vi "NI PXI Programmable Power Supply Ch Page.vi"(8 "error in (no error)":errorcluster, 11 "Node Ptr":T3 format="%.0x") -> (0 "error out":errorcluster)   [LabVIEW 2018, in "NI PXI-4110 Programmable Power Supply Custom Device.lvlib"]
uses:
  NI PXI-4110 Programmable Power Supply Custom Device.lvlib
  <vilib>/NI Veristand/Custom Device API/Custom Device Item Ref.ctl
  IO_Type.ctl
  4110_Channel #.ctl
  4110_Global.vi
  <vilib>/NI Veristand/Custom Device API/Get Item Property (Boolean).vi
  <vilib>/NI Veristand/Custom Device API/Get Item Property (U16).vi
  <vilib>/NI Veristand/Custom Device API/Get Item Property (Double).vi
  <vilib>/NI Veristand/Custom Device API/Set Item Property (U16).vi
  <vilib>/NI Veristand/Custom Device API/Set Item Property (Double).vi
  <vilib>/NI VeriStand/Custom Device API/Custom Device API.lvlib
panel:
  in  "Channel #":T1
  in  "Voltage Limit":dbl caption="Range (0-6V)" format="%.4f"
  in  "Initial Current Value":dbl caption="Range (0.01 -1A)" format="%.4f"
  in  "Current Limit":dbl caption="Range (0.01-1A)" format="%.4f"
  in  "IO Type":T2
  in  "Initial Voltage Value":dbl caption="Range (0-6V)" format="%_4f"
  in  "Name":string
  in  "Header":cluster{"Section Name":string}={"Section Name"="PXI-4110  Settings"}
  in  "Description":string
  # "Voltage  IO Settings"
  # "Current IO Settings"
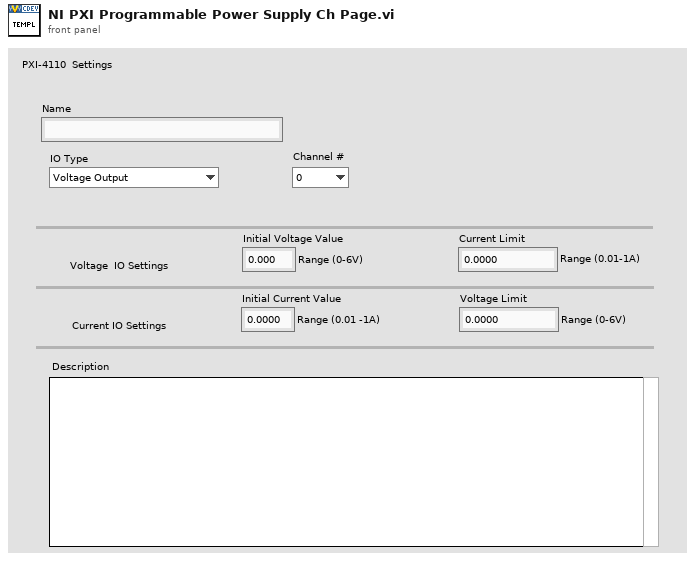
[diagram p1: front panel]
types:
  T1 = typedef "NI PXI-4110 Programmable Power Supply Custom Device.lvlib/4110_Channel #.ctl" = enum16{"0", "1", "2"}
  T2 = typedef "NI PXI-4110 Programmable Power Supply Custom Device.lvlib/IO_Type.ctl" = enum16{"Voltage Output", "Current Output"}
  T3 = typedef "Custom Device API.lvlib/Custom Device Item Ref.ctl" = u64
  T4 = cluster{"V_min":dbl, "V_max":dbl, "I_min":dbl, "I_max":dbl}
  T5 = enum8{"Enabled", "Disabled", "Disabled and Grayed Out"}
  T6 = typedef "Custom Device API.lvlib/Custom Device Item Info.ctl" = cluster{"Name":string, "Is Channel":bool, "GUID":string, "Is Waveform":bool}
  T7 = typedef "Custom Device API.lvlib/Custom Device Commands.ctl" = enum16{"Default", "Item renamed", "Shutdown", "Dynamic button pressed"}
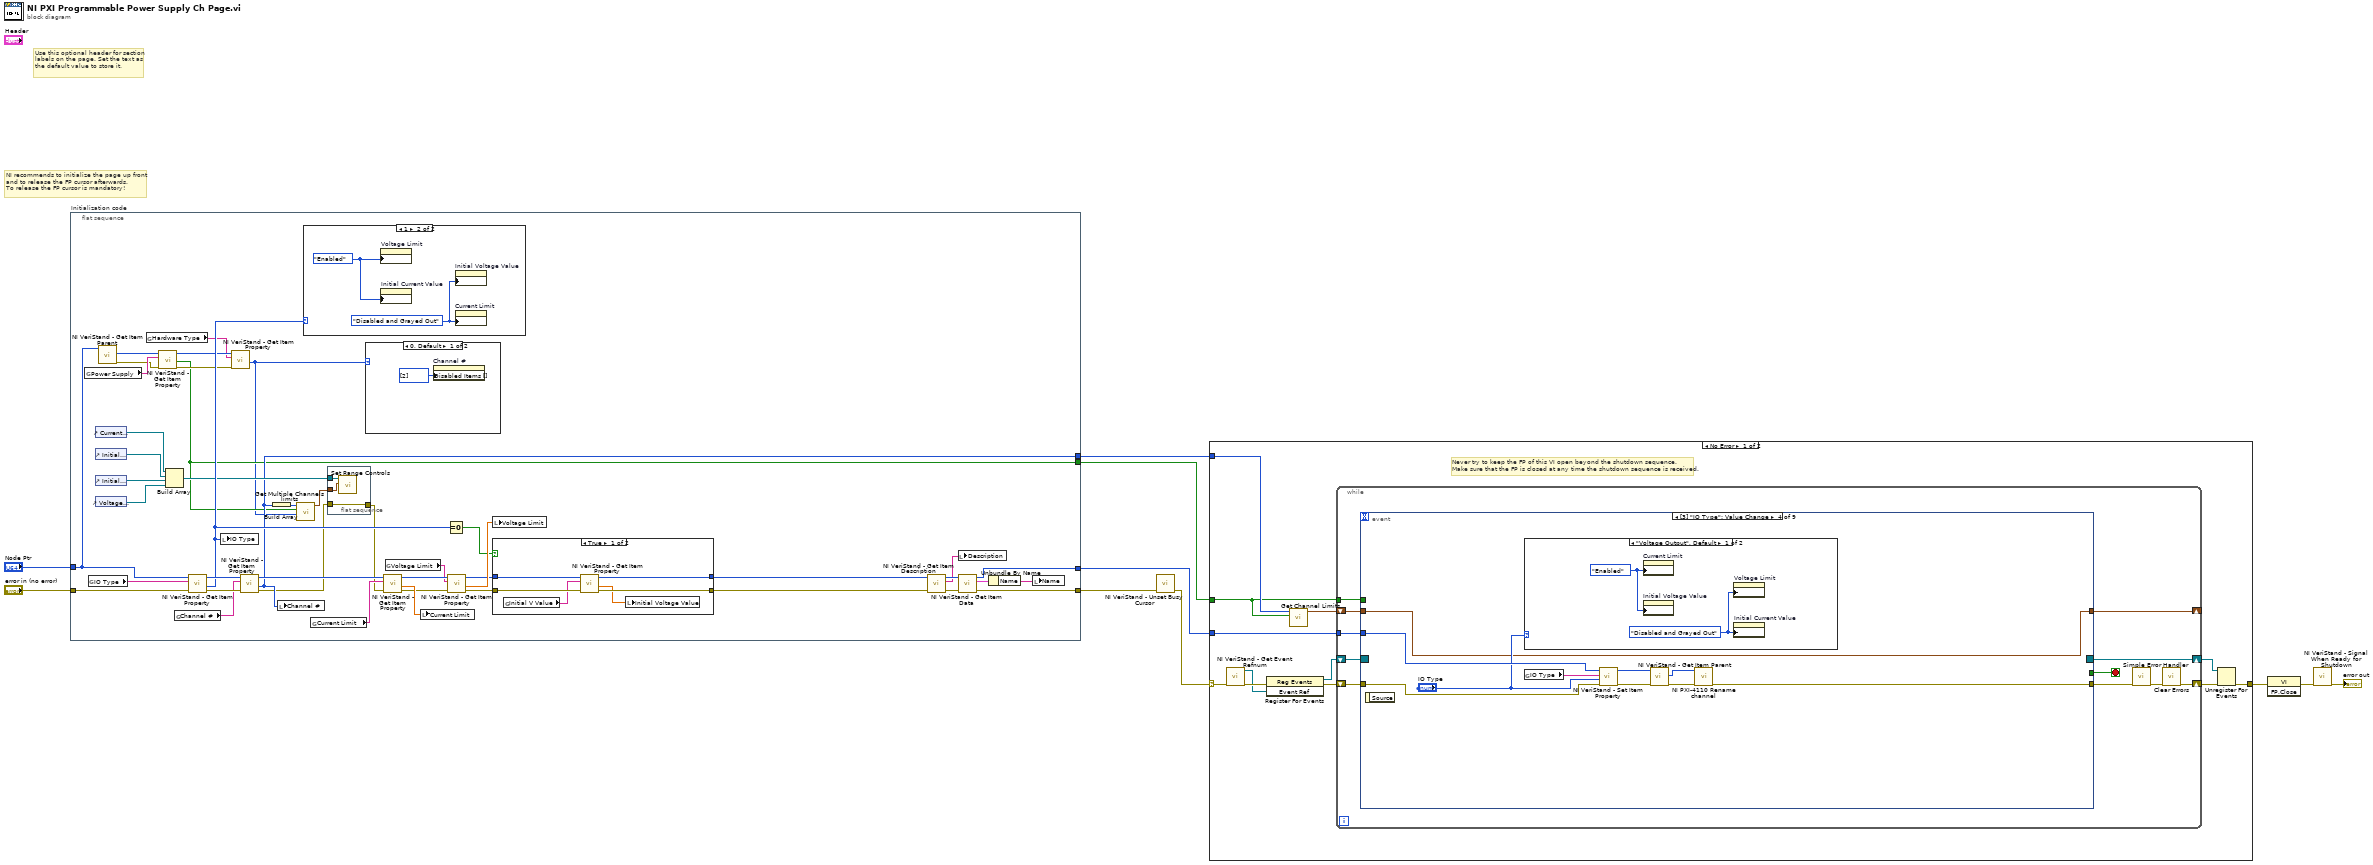
[diagram p0: block diagram]
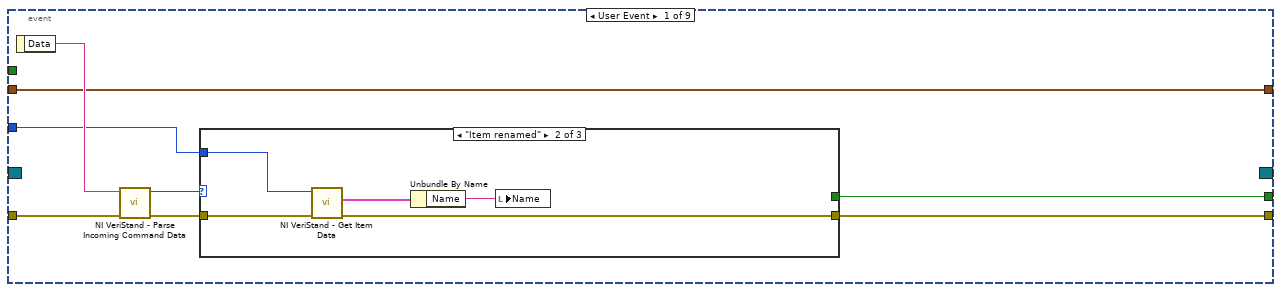
[diagram p2: hidden frame]
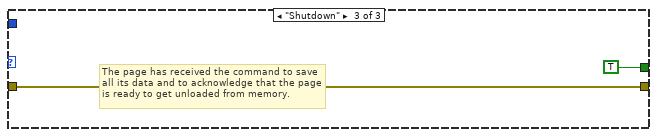
[diagram p4: hidden frame]
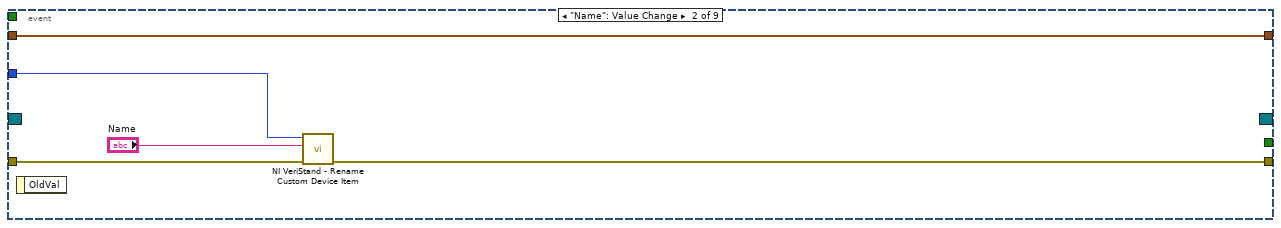
[diagram p5: hidden frame]
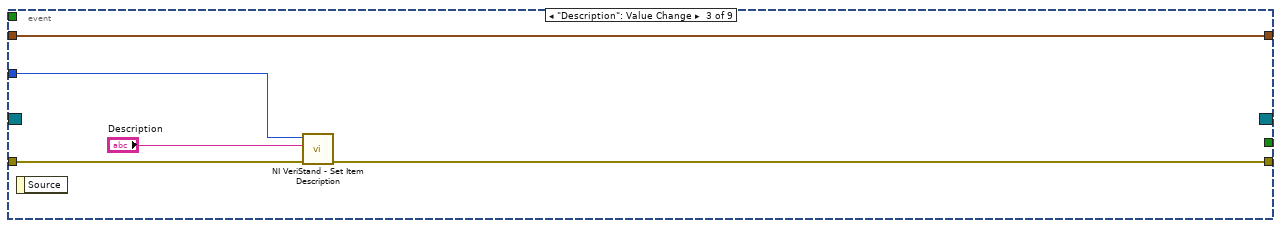
[diagram p6: hidden frame]
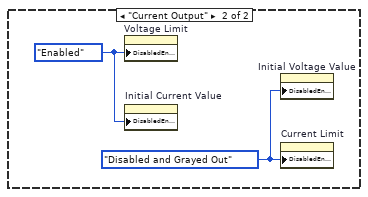
[diagram p7: hidden frame]
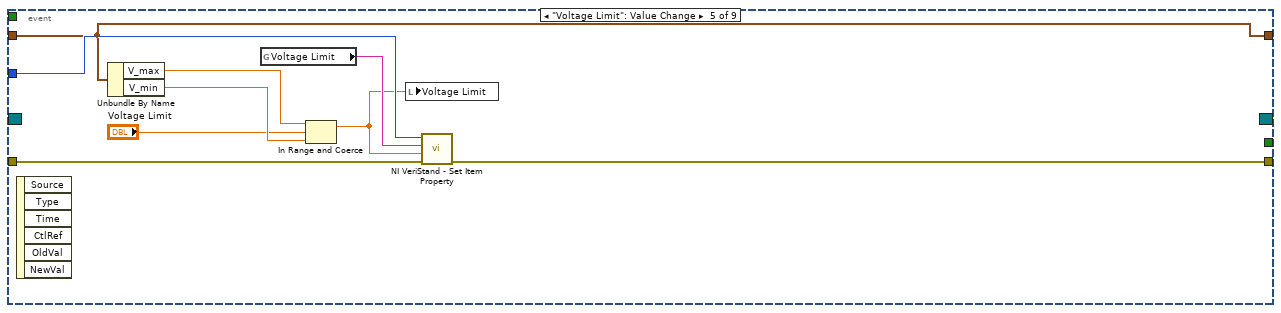
[diagram p8: hidden frame]
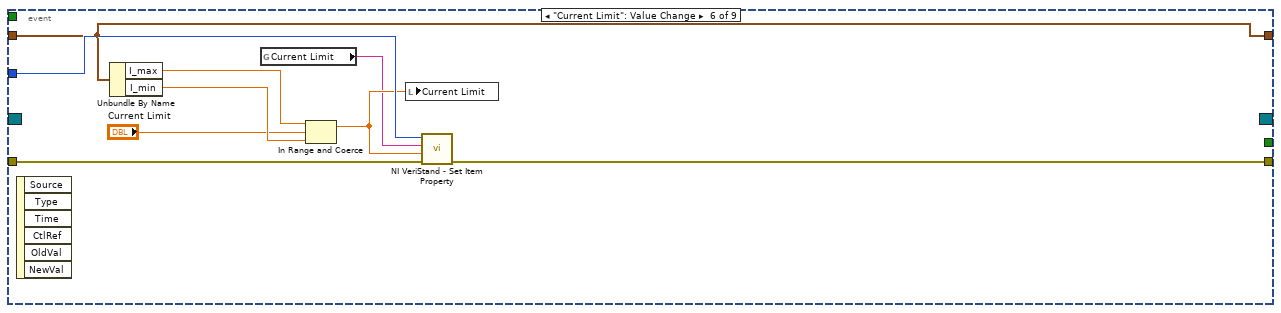
[diagram p9: hidden frame]
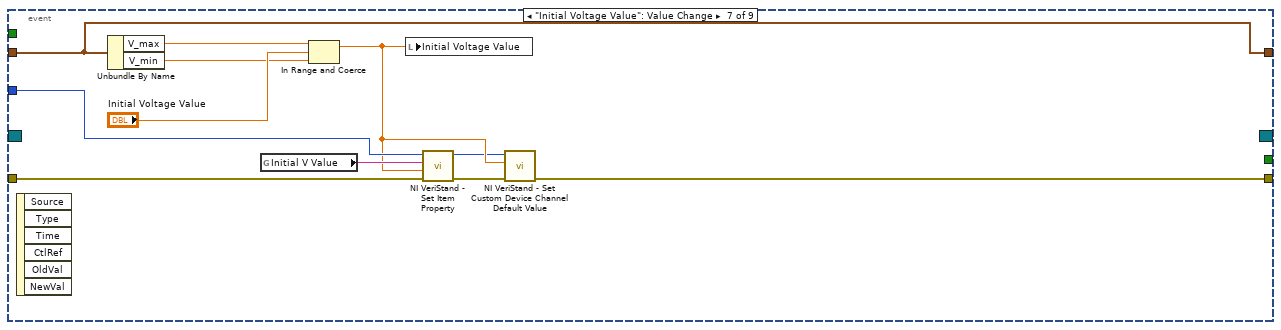
[diagram p10: hidden frame]
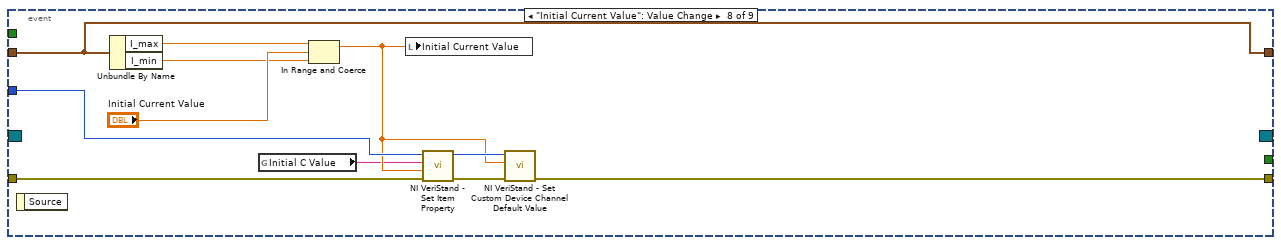
[diagram p11: hidden frame]
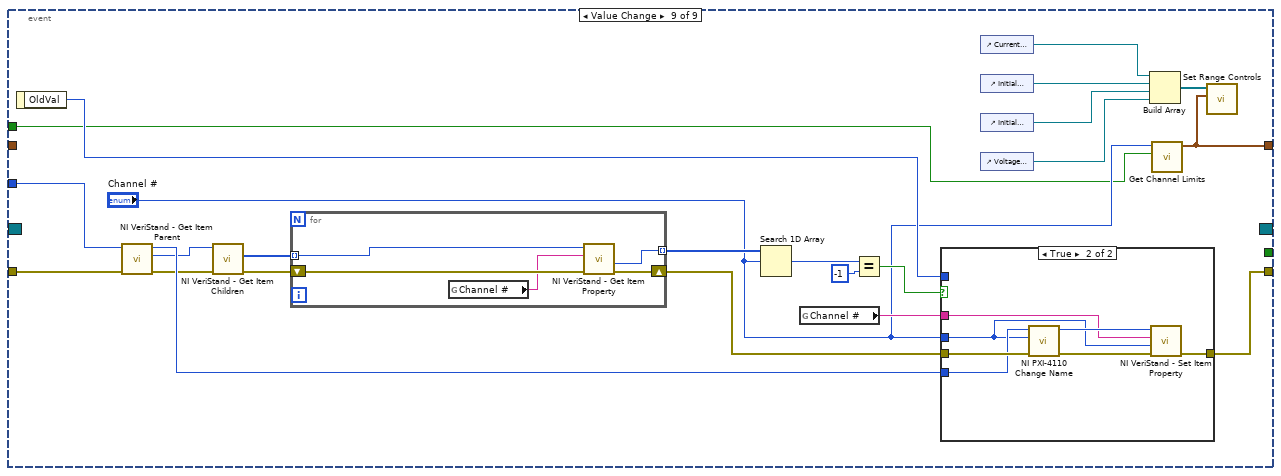
[diagram p12: hidden frame]
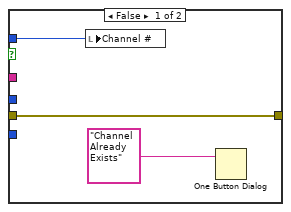
[diagram p13: hidden frame]
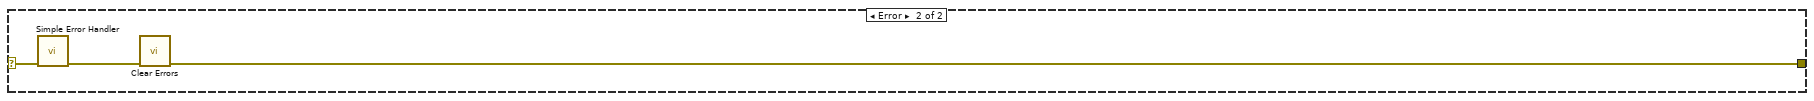
[diagram p14: hidden frame]
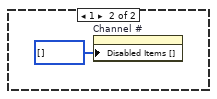
[diagram p15: hidden frame]
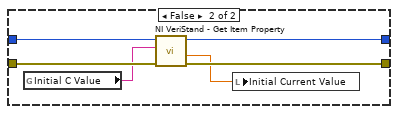
[diagram p16: hidden frame]
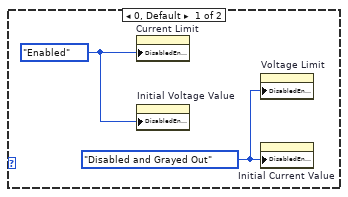
[diagram p17: hidden frame]
diagram:
  # "Use this optional header for section labels on the page. Set the text as the default value to store it."
  # "NI recommends to initialize the page up front\nand to release the FP cursor afterwards.\nTo release the FP cursor is mandatory!"
  n1 = flat-sequence "Initialization code" {
    tunnel: "error in (no error)" -> [w47]
    tunnel: "Node Ptr" -> [w31]
    tunnel: [w49] -> w6
    tunnel: [w54] -> w4
    tunnel: [w19] -> w2
    tunnel: [w17] -> w1
    frame #0 {
      n2 = global read "4110_Global.vi" "Power Supply"() -> (w30:string)
      n3 = global read "4110_Global.vi" "IO Type"() -> (w46:string)
      n4 = control-ref of="Current Limit"() -> (w24:refnum<vi>)
      n5 = control-ref of="Initial Current Value"() -> (w25:refnum<vi>)
      n6 = control-ref of="Initial Voltage Value"() -> (w26:refnum<vi>)
      n7 = control-ref of="Voltage Limit"() -> (w27:refnum<vi>)
      n8 = call <vilib>:"NI VeriStand - Get Item Parent.vi"("Item Ref in"=w31) -> ("error out"=w20:errorcluster, "Parent Ref"=w29:T3)  [unwired: 7 in, 2 out]
      n9 = global read "4110_Global.vi" "Hardware Type"() -> (w21:string)
      n10 = call-poly <vilib>:"NI VeriStand - Get Item Property.vi"("error in (no error)"=w20, "Property Name"=w30, "Item Ref in"=w29) -> ("error out"=w22:errorcluster, "Value"=w17:bool, "Item Ref out"=w23:T3)  [unwired: 5 in, 1 out]
      n11 = Build Array(w24, w25, w26, w27) -> (w28:refnum<vi>[])
      n12 = global read "4110_Global.vi" "Channel #"() -> (w43:string)
      n13 = call-poly <vilib>:"NI VeriStand - Get Item Property.vi"("error in (no error)"=w47, "Property Name"=w46, "Item Ref in"=w31) -> ("error out"=w45:errorcluster, "Value"=w33:u16, "Item Ref out"=w44:T3)  [unwired: 5 in, 1 out]
      n14 = local write "IO Type"(w33) -> ()
      n15 = call-poly <vilib>:"NI VeriStand - Get Item Property.vi"("error in (no error)"=w22, "Property Name"=w21, "Item Ref in"=w23) -> ("Value"=w16:u16)  [unwired: 5 in, 3 out]
      n16 = call-poly <vilib>:"NI VeriStand - Get Item Property.vi"("error in (no error)"=w45, "Property Name"=w43, "Item Ref in"=w44) -> ("error out"=w13:errorcluster, "Value"=w19:u16, "Item Ref out"=w42:T3)  [unwired: 5 in, 1 out]
      n17 = Build Array(w19) -> (w18:u16[])
      n18 = local write "Channel #"(w19) -> ()
      n19 = call "Get Multiple Channels limits.vi"("Power Supply In Use"=w16, "External Supply?"=w17, "Channels"=w18) -> ("output cluster"=w15:T4)  [unwired: 7 in, 1 out]
      n20 = case shown="1" w33 {
        frame 0, Default {
          w72 = T5."Enabled" ("Disabled")
          w73 = T5."Disabled and Grayed Out" ("Disabled")
          n21 = property on="Current Limit" class="DigNum (strict)"("DisabledEnum"=w72) -> ()  [unwired: 2 in, 2 out]
          n22 = property on="Initial Voltage Value" class="DigNum (strict)"("DisabledEnum"=w72) -> ()  [unwired: 2 in, 2 out]
          n23 = property on="Voltage Limit" class="DigNum (strict)"("DisabledEnum"=w73) -> ()  [unwired: 2 in, 2 out]
          n24 = property on="Initial Current Value" class="DigNum (strict)"("DisabledEnum"=w73) -> ()  [unwired: 2 in, 2 out]
        }
        frame 1 {
          w74 = T5."Enabled" ("Disabled")
          w75 = T5."Disabled and Grayed Out" ("Disabled")
          n25 = property on="Voltage Limit" class="DigNum (strict)"("DisabledEnum"=w74) -> ()  [unwired: 2 in, 2 out]
          n26 = property on="Initial Current Value" class="DigNum (strict)"("DisabledEnum"=w74) -> ()  [unwired: 2 in, 2 out]
          n27 = property on="Initial Voltage Value" class="DigNum (strict)"("DisabledEnum"=w75) -> ()  [unwired: 2 in, 2 out]
          n28 = property on="Current Limit" class="DigNum (strict)"("DisabledEnum"=w75) -> ()  [unwired: 2 in, 2 out]
        }
      }
      n29 = global read "4110_Global.vi" "Current Limit"() -> (w41:string)
      n30 = flat-sequence {
        tunnel: w28 -> [w57]
        tunnel: w15 -> [w56]
        tunnel: [w55] -> w14
        tunnel: w13 -> [w55]
        frame #0 {
          n31 = call "Set Range Controls.vi"("Ranges"=w56, "Reference Array"=w57) -> ()  [unwired: 10 in]
        }
      }
      n32 = case shown="0, Default" w16 {
        frame 0, Default {
          n33 = property on="Channel #" class="Enum (strict)"("Disabled Items []"=i32[] [2]) -> ()  [unwired: 2 in, 2 out]
        }
        frame 1 {
          n34 = property on="Channel #" class="Enum (strict)"("Disabled Items []"=i32[] []) -> ()  [unwired: 2 in, 2 out]
        }
      }
      n35 = call-poly <vilib>:"NI VeriStand - Get Item Property.vi"("error in (no error)"=w14, "Property Name"=w41, "Item Ref in"=w42) -> ("error out"=w39:errorcluster, "Value"=w40:dbl, "Item Ref out"=w38:T3)  [unwired: 5 in, 1 out]
      n36 = global read "4110_Global.vi" "Voltage Limit"() -> (w37:string)
      n37 = local write "Current Limit"(w40) -> ()
      n38 = Equal To 0?(x=w33) -> (x = 0?=w32:bool)
      n39 = call-poly <vilib>:"NI VeriStand - Get Item Property.vi"("error in (no error)"=w39, "Property Name"=w37, "Item Ref in"=w38) -> ("error out"=w34:errorcluster, "Value"=w36:dbl, "Item Ref out"=w35:T3)  [unwired: 5 in, 1 out]
      n40 = local write "Voltage Limit"(w36) -> ()
      n41 = case shown="True" w32 {
        tunnel: w35 -> [w65 w71]
        tunnel: w34 -> [w64 w70]
        tunnel: [w63 w69] -> w11
        tunnel: [w62 w68] -> w12
        frame True {
          n42 = global read "4110_Global.vi" "Initial V Value"() -> (w61:string)
          n43 = call-poly <vilib>:"NI VeriStand - Get Item Property.vi"("error in (no error)"=w64, "Property Name"=w61, "Item Ref in"=w65) -> ("error out"=w63:errorcluster, "Value"=w60:dbl, "Item Ref out"=w62:T3)  [unwired: 5 in, 1 out]
          n44 = local write "Initial Voltage Value"(w60) -> ()
        }
        frame False {
          n45 = global read "4110_Global.vi" "Initial C Value"() -> (w67:string)
          n46 = call-poly <vilib>:"NI VeriStand - Get Item Property.vi"("error in (no error)"=w70, "Property Name"=w67, "Item Ref in"=w71) -> ("error out"=w69:errorcluster, "Value"=w66:dbl, "Item Ref out"=w68:T3)  [unwired: 5 in, 1 out]
          n47 = local write "Initial Current Value"(w66) -> ()
        }
      }
      n48 = call <vilib>:"NI VeriStand - Get Item Description.vi"("error in (no error)"=w11, "Item Ref in"=w12) -> ("error out"=w51:errorcluster, "Description"=w52:string, "Item Ref out"=w53:T3)  [unwired: 7 out]
      n49 = local write "Description"(w52) -> ()
      n50 = call <vilib>:"NI VeriStand - Get Item Data.vi"("error in (no error)"=w51, "Item Ref in"=w53) -> ("error out"=w49:errorcluster, "Item Info"=w50:T6, "Item Ref out"=w54:T3)  [unwired: 7 out]
      n51 = Unbundle By Name(w50) -> ("Name"=w48:string)
      n52 = local write "Name"(w48) -> ()
    }
  }
  n53 = call <vilib>:"NI VeriStand - Unset Busy Cursor.vi"("error in (no error)"=w6) -> ("error out"=w5:errorcluster)  [unwired: 10 out]
  n54 = case shown="No Error" w5 {
    selector: w5 -> [w79 w219]
    tunnel: [w84 w217] -> w10
    tunnel: w4 -> [w80 _]
    tunnel: w2 -> [w78 _]
    tunnel: w1 -> [w76 _]
    frame No Error {
      # "Never try to keep the FP of this VI open beyond the shutdown sequence.\nMake sure that the FP is closed at any time the shutdown sequence is received."
      n55 = call <vilib>:"NI VeriStand - Get Event Refnum.vi"("error in (no error)"=w79) -> ("error out"=w87:errorcluster, "Event Ref"=w83:refnum<user-event>)  [unwired: 9 out]
      n56 = register-events(error in=w87, w83) -> (reference out=w81:refnum<event-registration>, error out=w82:errorcluster)  [unwired: 1 in]
      n57 = call "Get Channel Limits.vi"("External Supply?"=w76, "Channel #"=w78) -> ("output cluster"=w77:T4)  [unwired: 8 in, 1 out]
      n58 = while {
        tunnel: w80 -> [w94]
        shift-right: [w91] -> w85
        shift-left: w82 -> [w97]
        shift-right: [w98] -> w86
        shift-left: w81 -> [w96]
        shift-right: [w90] -> _
        shift-left: w77 -> [w89]
        tunnel: w76 -> [w88]
        stop <- w95 stop-if-true
        n59 = event shown="[3] \"IO Type\": Value Change" {
          selector: w96 -> [_ _ _ _ _ _ _ _ _]
          dyn-events: [_ _ _ _ _ _ _ _ _] -> w98
          timeout: _ -> [_ _ _ _ _ _ _ _ _]
          tunnel: w97 -> [w106 w119 w123 w133 w146 w155 w166 w177 w188]
          tunnel: [w102 _ _ _ _ _ _ _ _] -> w95
          tunnel: [w101 w118 w122 w128 w145 w154 w163 w175 w187] -> w93
          tunnel: w94 -> [w100 w117 w124 w134 w147 w156 w167 w178 w189]
          tunnel: [w99 w115 w120 w126 w143 w151 w159 w172 w179] -> w90
          tunnel: w89 -> [w99 w115 w120 w126 w143 w151 w159 w172 _]
          tunnel: w88 -> [_ _ _ _ _ _ _ _ w185]
          event User Event {
            n60 = event-data() -> ("Data"=w105:string)  [unwired: 1 out]
            n61 = call <vilib>:"NI VeriStand - Parse Incoming Command Data.vi"("error in (no error)"=w106, "Incoming data"=w105) -> ("error out"=w104:errorcluster, "Action"=w103:T7)  [unwired: 8 out]
            n62 = case shown="\"Item renamed\"" w103 {
              tunnel: w104 -> [w107 w112 w113]
              tunnel: [_ _ TRUE] -> w102
              tunnel: [w107 w109 w113] -> w101
              tunnel: w100 -> [_ w111 _]
              frame "Default", Default {
              }
              frame "Item renamed" {
                n63 = call <vilib>:"NI VeriStand - Get Item Data.vi"("error in (no error)"=w112, "Item Ref in"=w111) -> ("error out"=w109:errorcluster, "Item Info"=w110:T6)  [unwired: 8 out]
                n64 = Unbundle By Name(w110) -> ("Name"=w108:string)
                n65 = local write "Name"(w108) -> ()
              }
              frame "Shutdown" {
                # "The page has received the command to save all its data and to acknowledge that the page is ready to get unloaded from memory."
              }
            }
          }
          event "Name": Value Change {
            n66 = event-data() -> ()  [unwired: 2 out]
            n67 = call <vilib>:"NI VeriStand - Rename Custom Device Item.vi"("error in (no error)"=w119, "New Name"="Name", "Item Ref in"=w117) -> ("error out"=w118:errorcluster)  [unwired: 1 in, 7 out]
          }
          event "Description": Value Change {
            n68 = event-data() -> ()  [unwired: 2 out]
            n69 = call <vilib>:"NI VeriStand - Set Item Description.vi"("error in (no error)"=w123, "Description"="Description", "Item Ref in"=w124) -> ("error out"=w122:errorcluster)  [unwired: 8 out]
          }
          event Value Change {
            n70 = event-data() -> ()  [unwired: 2 out]
            n71 = case shown="\"Voltage Output\", Default" "IO Type" {
              frame "Voltage Output", Default {
                w135 = T5."Enabled" ("Disabled")
                w136 = T5."Disabled and Grayed Out" ("Disabled")
                n72 = property on="Current Limit" class="DigNum (strict)"("DisabledEnum"=w135) -> ()  [unwired: 2 in, 2 out]
                n73 = property on="Initial Voltage Value" class="DigNum (strict)"("DisabledEnum"=w135) -> ()  [unwired: 2 in, 2 out]
                n74 = property on="Voltage Limit" class="DigNum (strict)"("DisabledEnum"=w136) -> ()  [unwired: 2 in, 2 out]
                n75 = property on="Initial Current Value" class="DigNum (strict)"("DisabledEnum"=w136) -> ()  [unwired: 2 in, 2 out]
              }
              frame "Current Output" {
                w137 = T5."Enabled" ("Disabled")
                w138 = T5."Disabled and Grayed Out" ("Disabled")
                n76 = property on="Voltage Limit" class="DigNum (strict)"("DisabledEnum"=w137) -> ()  [unwired: 2 in, 2 out]
                n77 = property on="Initial Current Value" class="DigNum (strict)"("DisabledEnum"=w137) -> ()  [unwired: 2 in, 2 out]
                n78 = property on="Initial Voltage Value" class="DigNum (strict)"("DisabledEnum"=w138) -> ()  [unwired: 2 in, 2 out]
                n79 = property on="Current Limit" class="DigNum (strict)"("DisabledEnum"=w138) -> ()  [unwired: 2 in, 2 out]
              }
            }
            n80 = global read "4110_Global.vi" "IO Type"() -> (w132:string)
            n81 = call-poly <vilib>:"NI VeriStand - Set Item Property.vi"("error in (no error)"=w133, "Value"="IO Type", "Property Name"=w132, "Item Ref in"=w134) -> ("error out"=w130:errorcluster, "Item Ref out"=w129:T3)  [unwired: 5 in, 1 out]
            n82 = call <vilib>:"NI VeriStand - Get Item Parent.vi"("error in (no error)"=w130, "Item Ref in"=w129) -> ("error out"=w127:errorcluster, "Parent Ref"=w125:T3)  [unwired: 6 in, 2 out]
            n83 = call "NI PXI-4110 Rename channel.vi"("error in (no error)"=w127, "Section Ptr"=w125) -> ("error out"=w128:errorcluster)  [unwired: 8 in, 1 out]
          }
          event "Voltage Limit": Value Change {
            n84 = event-data() -> ()  [unwired: 7 out]
            n85 = Unbundle By Name(w143) -> ("V_max"=w142:dbl, "V_min"=w141:dbl)
            n86 = global read "4110_Global.vi" "Voltage Limit"() -> (w144:string)
            n87 = In Range and Coerce(upper limit=w142, x="Voltage Limit", lower limit=w141) -> (coerced(x)=w139:dbl)  [unwired: 1 out]
            n88 = local write "Voltage Limit"(w139) -> ()
            n89 = call-poly <vilib>:"NI VeriStand - Set Item Property.vi"("error in (no error)"=w146, "Value"=w139, "Property Name"=w144, "Item Ref in"=w147) -> ("error out"=w145:errorcluster)  [unwired: 5 in, 2 out]
          }
          event "Current Limit": Value Change {
            n90 = event-data() -> ()  [unwired: 7 out]
            n91 = Unbundle By Name(w151) -> ("I_max"=w153:dbl, "I_min"=w152:dbl)
            n92 = global read "4110_Global.vi" "Current Limit"() -> (w148:string)
            n93 = In Range and Coerce(upper limit=w153, x="Current Limit", lower limit=w152) -> (coerced(x)=w149:dbl)  [unwired: 1 out]
            n94 = local write "Current Limit"(w149) -> ()
            n95 = call-poly <vilib>:"NI VeriStand - Set Item Property.vi"("error in (no error)"=w155, "Value"=w149, "Property Name"=w148, "Item Ref in"=w156) -> ("error out"=w154:errorcluster)  [unwired: 5 in, 2 out]
          }
          event "Initial Voltage Value": Value Change {
            n96 = event-data() -> ()  [unwired: 7 out]
            n97 = Unbundle By Name(w159) -> ("V_max"=w158:dbl, "V_min"=w157:dbl)
            n98 = global read "4110_Global.vi" "Initial V Value"() -> (w165:string)
            n99 = In Range and Coerce(upper limit=w158, x="Initial Voltage Value", lower limit=w157) -> (coerced(x)=w162:dbl)  [unwired: 1 out]
            n100 = local write "Initial Voltage Value"(w162) -> ()
            n101 = call-poly <vilib>:"NI VeriStand - Set Item Property.vi"("error in (no error)"=w166, "Value"=w162, "Property Name"=w165, "Item Ref in"=w167) -> ("error out"=w164:errorcluster, "Item Ref out"=w161:T3)  [unwired: 5 in, 1 out]
            n102 = call <vilib>:"NI VeriStand - Set Custom Device Channel Default Value.vi"("error in (no error)"=w164, "Default Value"=w162, "Channel Ref in"=w161) -> ("error out"=w163:errorcluster)  [unwired: 7 in, 1 out]
          }
          event "Initial Current Value": Value Change {
            n103 = event-data() -> ()  [unwired: 2 out]
            n104 = Unbundle By Name(w172) -> ("I_max"=w171:dbl, "I_min"=w170:dbl)
            n105 = global read "4110_Global.vi" "Initial C Value"() -> (w168:string)
            n106 = In Range and Coerce(upper limit=w171, x="Initial Current Value", lower limit=w170) -> (coerced(x)=w169:dbl)  [unwired: 1 out]
            n107 = local write "Initial Current Value"(w169) -> ()
            n108 = call-poly <vilib>:"NI VeriStand - Set Item Property.vi"("error in (no error)"=w177, "Value"=w169, "Property Name"=w168, "Item Ref in"=w178) -> ("error out"=w176:errorcluster, "Item Ref out"=w174:T3)  [unwired: 5 in, 1 out]
            n109 = call <vilib>:"NI VeriStand - Set Custom Device Channel Default Value.vi"("error in (no error)"=w176, "Default Value"=w169, "Channel Ref in"=w174) -> ("error out"=w175:errorcluster)  [unwired: 7 in, 1 out]
          }
          event Value Change {
            n110 = event-data() -> ("OldVal"=w191:T1)  [unwired: 1 out]
            n111 = call <vilib>:"NI VeriStand - Get Item Parent.vi"("error in (no error)"=w188, "Item Ref in"=w189) -> ("error out"=w192:errorcluster, "Parent Ref"=w193:T3, "Item Ref out"=w201:T3)  [unwired: 6 in, 1 out]
            n112 = call <vilib>:"NI VeriStand - Get Item Children.vi"("error in (no error)"=w192, "Item Ref in"=w193) -> ("error out"=w195:errorcluster, "Child Refs"=w194:T3[])  [unwired: 6 in, 2 out]
            n113 = for {
              tunnel: w194 -> [w214] mode=indexing
              shift-right: [w215] -> w200
              shift-left: w195 -> [w216]
              tunnel: [w213] -> w196 mode=indexing
              n114 = global read "4110_Global.vi" "Channel #"() -> (w212:string)
              n115 = call-poly <vilib>:"NI VeriStand - Get Item Property.vi"("error in (no error)"=w216, "Property Name"=w212, "Item Ref in"=w214) -> ("error out"=w215:errorcluster, "Value"=w213:u16)  [unwired: 5 in, 2 out]
            }
            n116 = Search 1D Array(1D array=w196, element="Channel #") -> (index of element=w197:i32)  [unwired: 1 in]
            n117 = global read "4110_Global.vi" "Channel #"() -> (w190:string)
            n118 = Equal?(x=w197, y=-1) -> (x = y?=w199:bool)
            n119 = case shown="True" w199 {
              tunnel: w200 -> [w203 w211]
              tunnel: w201 -> [_ w210]
              tunnel: w190 -> [_ w206]
              tunnel: "Channel #" -> [_ w205]
              tunnel: [w203 w208] -> w187
              tunnel: w191 -> [w204 _]
              frame False {
                n120 = local write "Channel #"(w204) -> ()
                n121 = One Button Dialog(message="Channel Already Exists") -> ()  [unwired: 1 in, 1 out]
              }
              frame True {
                n122 = call "NI PXI-4110 Change Name.vi"("error in (no error)"=w211, "New #"=w205, "Node Ptr"=w210) -> ("error out"=w209:errorcluster, "Node Ptr out"=w207:T3)  [unwired: 7 in]
                n123 = call-poly <vilib>:"NI VeriStand - Set Item Property.vi"("error in (no error)"=w209, "Value"=w205, "Property Name"=w206, "Item Ref in"=w207) -> ("error out"=w208:errorcluster)  [unwired: 5 in, 2 out]
              }
            }
            n124 = control-ref of="Current Limit"() -> (w184:refnum<vi>)
            n125 = control-ref of="Initial Current Value"() -> (w183:refnum<vi>)
            n126 = control-ref of="Initial Voltage Value"() -> (w182:refnum<vi>)
            n127 = control-ref of="Voltage Limit"() -> (w181:refnum<vi>)
            n128 = Build Array(w184, w183, w182, w181) -> (w180:refnum<vi>[])
            n129 = call "Get Channel Limits.vi"("External Supply?"=w185, "Channel #"="Channel #") -> ("output cluster"=w179:T4)  [unwired: 8 in, 1 out]
            n130 = call "Set Range Controls.vi"("Ranges"=w179, "Reference Array"=w180) -> ()  [unwired: 10 in]
          }
        }
        n131 = call <vilib>:"Simple Error Handler.vi"("error in (no error)"=w93) -> ("error out"=w92:errorcluster)  [unwired: 1 in, 7 out]
        n132 = call <vilib>:"Clear Errors.vi"("error in (no error)"=w92) -> ("error out"=w91:errorcluster)  [unwired: 1 in, 5 out]
      }
      n133 = Unregister For Events(event registration refnum=w86, error in=w85) -> (error out=w84:errorcluster)
    }
    frame Error {
      n134 = call <vilib>:"Simple Error Handler.vi"("error in (no error)"=w219) -> ("error out"=w218:errorcluster)  [unwired: 1 in, 7 out]
      n135 = call <vilib>:"Clear Errors.vi"("error in (no error)"=w218) -> ("error out"=w217:errorcluster)  [unwired: 1 in, 5 out]
    }
  }
  n136 = invoke class="VI" method="FP.Close"(error in=w10) -> (error out=w9:errorcluster)  [unwired: 2 in, 2 out]
  n137 = call <vilib>:"NI VeriStand - Signal When Ready for Shutdown.vi"("error in (no error)"=w9) -> ("error out"=→"error out":errorcluster)  [unwired: 10 out]
